vi "Status Reference.vi"(0 "Test in":refnum<class "Test.lvclass">, 11 "Error in":errorcluster) -> (4 "Test out":refnum<class "Test.lvclass">, 6 "VI ref":refnum<vi>, 15 "Error out":errorcluster)   [LabVIEW 2020, in "Test.lvclass"]
doc: "Dynamic method for status page reference"
uses:
  Test.lvclass
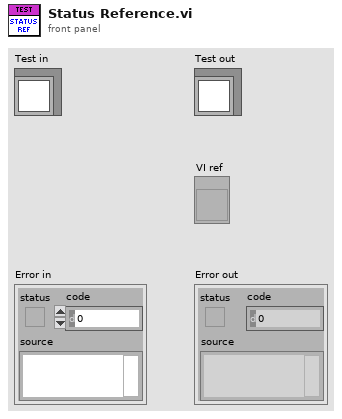
[diagram p1: front panel]
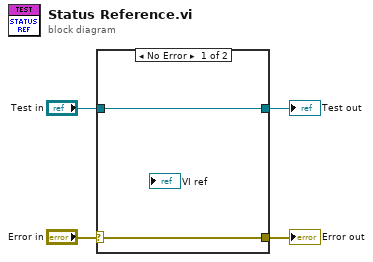
[diagram p0: block diagram]
diagram:
  n1 = case shown="No Error" "Error in" {
    selector: "Error in" -> [w5 w8]
    tunnel: [w5 w8] -> w3
    tunnel: [w6 w7] -> w1
    tunnel: "Test in" -> [w6 w7]
    frame No Error {
    }
    frame Error {
    }
  }
  "Error out" <- w3
  "Test out" <- w1
